vi "Configurações.vi"(8 "error in (no error)":errorcluster, 9 "Configurações":T1={"Simulações"={"Nível Qualidade"="avi", "Turno"="avi"}, "Captura de Imagens"={"Pasta com imagens"=path "", "Mostrar imagens capturadas"=FALSE}, "Caminhos"={"Arquivo de configuração"=path ""}}, 11 "Ação":T2) -> (0 "error out":errorcluster, 1 "Configurações Salvas":T1={"Simulações"={"Nível Qualidade"="avi", "Turno"="avi"}, "Captura de Imagens"={"Pasta com imagens"=path "", "Mostrar imagens capturadas"=FALSE}, "Caminhos"={"Arquivo de configuração"=path ""}})   [LabVIEW 2020, in "Configurações.lvlib"]
doc: "Gerenciador de configurações\nPara adicionar ou alterar mais opções de configuração, altere o Type Def \"Configurações Padrões.ctl\""
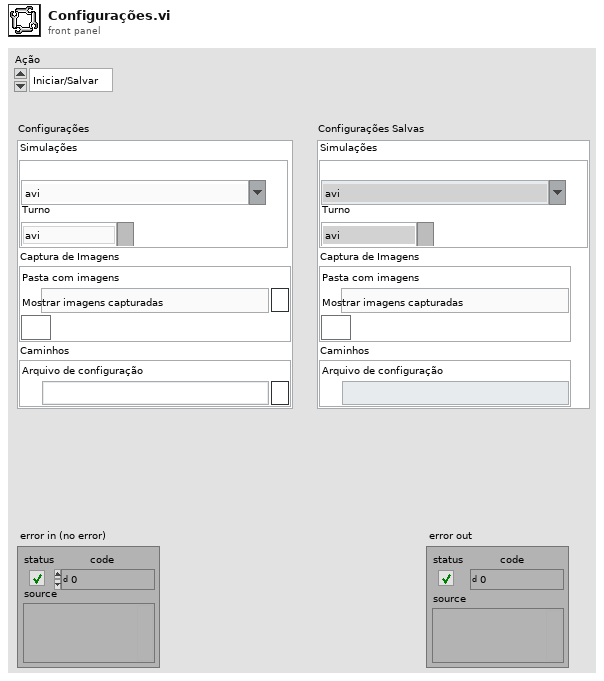
[diagram p1: front panel]
types:
  T1 = typedef "Configurações.lvlib/Configurações padrões.ctl" = cluster{"Simulações":cluster{"Nível Qualidade":string, "Turno":string}, "Captura de Imagens":cluster{"Pasta com imagens":path, "Mostrar imagens capturadas":bool}, "Caminhos":cluster{"Arquivo de configuração":path}}
  T2 = typedef "Ações de configuração.ctl" = enum16{"Iniciar/Salvar", "Ler"}
  T3 = typedef "Ações de configuração 2.ctl" = enum16{"Escrita", "Leitura"}
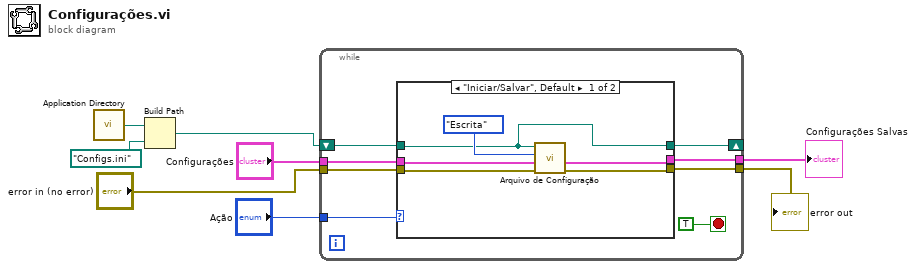
[diagram p0: block diagram]
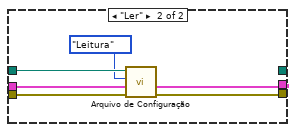
[diagram p2: hidden frame]
diagram:
  n1 = call <vilib>:"Application Directory.vi"() -> ("Application Directory"=w6:path)
  n2 = Build Path(base path=w6, name or relative path=path "Configs.ini") -> (appended path=w4:path)
  n3 = while {
    tunnel: "Ação" -> [w16]
    tunnel: "Configurações" -> [w15]
    shift-right: [w14] -> _
    shift-left: w4 -> [w12]
    tunnel: "error in (no error)" -> [w11]
    tunnel: [w10] -> w2
    tunnel: [w9] -> w1
    stop <- TRUE stop-if-true
    n4 = case shown="\"Iniciar/Salvar\", Default" w16 {
      tunnel: w15 -> [w21 w26]
      tunnel: [w20 _] -> w14
      tunnel: w12 -> [w20 w28]
      tunnel: w11 -> [w19 w25]
      tunnel: [w18 w24] -> w10
      tunnel: [w17 w23] -> w9
      frame "Iniciar/Salvar", Default {
        n5 = call "Arquivo de Configuração.vi"("Caminho do arquivo"=w20, "Modo"=Ações_de_configuração_2."Escrita", "Configurações"=w21, "error in (no error)"=w19) -> ("Configurações 2"=w17:T1, "error out"=w18:errorcluster)  [unwired: 5 in]
      }
      frame "Ler" {
        n6 = call "Arquivo de Configuração.vi"("Caminho do arquivo"=w28, "Modo"=Ações_de_configuração_2."Leitura", "Configurações"=w26, "error in (no error)"=w25) -> ("Configurações 2"=w23:T1, "error out"=w24:errorcluster)  [unwired: 5 in]
      }
    }
  }
  "error out" <- w2
  "Configurações Salvas" <- w1
